vi "FlattenFRF.vi"(9 "CrsrList":T1, 11 "Complex FRF in":cluster{"t0":dbl, "dt":dbl, "Y":cdb[]}) -> (1 "Complex FRF out":cluster{"t0":dbl, "dt":dbl, "Y":cdb[]})   [LabVIEW 2022 SP3]
uses:
  <vilib>/Utility/miscctls.llb/LVCursorListTypeDef.ctl
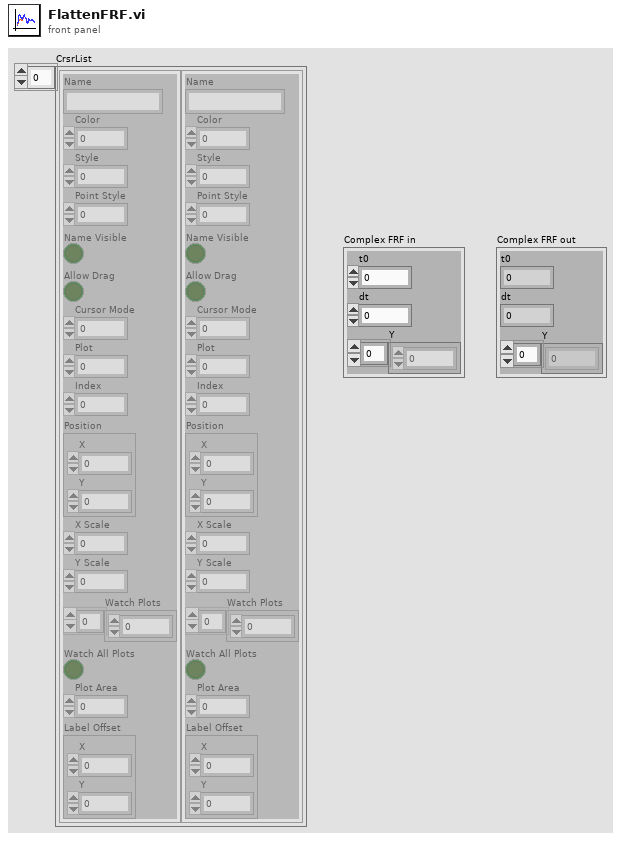
[diagram p1: front panel]
types:
  T1 = typedef "LVCursorListTypeDef.ctl" = cluster{"Name":string, "Color":u32, "Style":u8, "Point Style":u8, "Name Visible":bool, "Allow Drag":bool, "Cursor Mode":u32, "Plot":i32, "Index":i32, "Position":cluster{"X":dbl, "Y":dbl}, "X Scale":u32, "Y Scale":u32, "Watch Plots":i32[], "Watch All Plots":bool, "Plot Area":i32, "Label Offset":cluster{"X":dbl, "Y":dbl}}[]
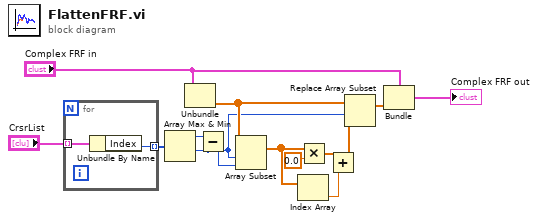
[diagram p0: block diagram]
diagram:
  n1 = for {
    tunnel: "CrsrList" -> [w16] mode=indexing
    tunnel: [w15] -> w9 mode=indexing
    n2 = Unbundle By Name(w16) -> ("Index"=w15:i32)
  }
  n3 = Array Max & Min(array=w9) -> (max value=w6:i32, min value=w7:i32)  [unwired: 2 out]
  n4 = Unbundle("Complex FRF in") -> ("Y"=w8:cdb[])  [unwired: 2 out]
  n5 = Subtract(x=w6, y=w7) -> (x-y=w5:i32)
  n6 = Array Subset(array=w8, index=w7, length=w5) -> (w3:cdb[])
  n7 = Index Array(array=w3) -> (element=w2:cdb)  [unwired: 1 in]
  n8 = Multiply(x=w3, y=0.0) -> (x*y=w4:cdb[])
  n9 = Add(x=w4, y=w2) -> (x+y=w1:cdb[])
  n10 = Replace Array Subset(array=w8, new element=w1, index=w7) -> (w10:cdb[])
  n11 = Bundle(cluster="Complex FRF in", "Y"=w10) -> (→"Complex FRF out":cluster{"t0":dbl, "dt":dbl, "Y":cdb[]})  [unwired: 2 in]
